vi "PathToQuotedString.vi"(10 "Path":path) -> (2 "String":string)   [LabVIEW 2023]
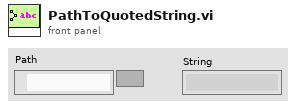
[diagram p1: front panel]
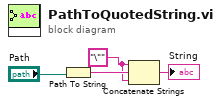
[diagram p0: block diagram]
diagram:
  w2 = "\"" ("string")
  n1 = Path To String(path="Path") -> (string=w3:string)
  n2 = Concatenate Strings(w2, w3, w2) -> (→"String":string)
